vi "1.vi"() -> ()   [LabVIEW 2015]
uses:
  <vilib>/Analysis/NI_AALBase.lvlib
panel:
  out "Simulasi Data":dbl[][](graph)
  in  "UUT Serial Number":string
  in  "Operator Name":string
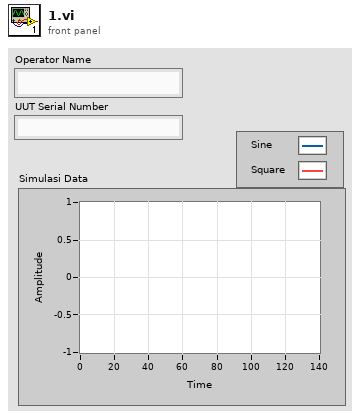
[diagram p1: front panel]
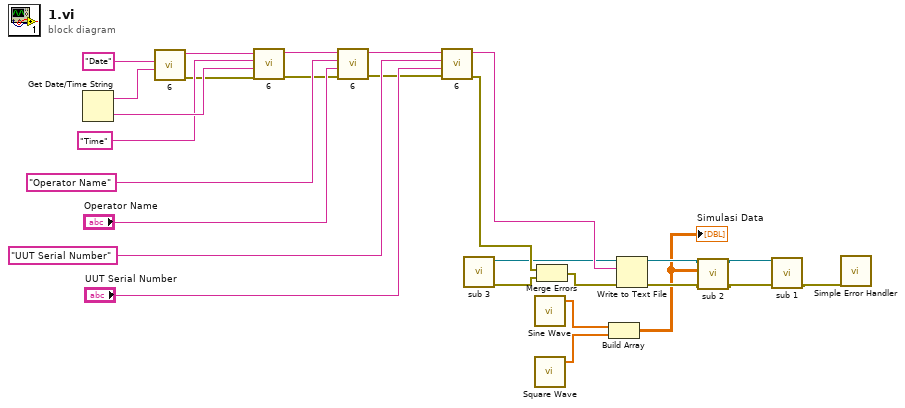
[diagram p0: block diagram]
diagram:
  n1 = Get Date/Time String() -> (date string=w9:string, time string=w8:string)  [unwired: 3 in]
  n2 = call "6.vi"(9:"File Property Name"=w9, 10:"File Property Name"="Date" ("input in")) -> ("error out"=w6:errorcluster, "String out"=w5:string)  [unwired: 8 in]
  n3 = call "6.vi"("error in (no error)"=w6, 9:"File Property Name"=w8, 10:"File Property Name"="Time" ("input in"), "String in"=w5) -> ("error out"=w4:errorcluster, "String out"=w3:string)  [unwired: 6 in]
  n4 = call "6.vi"("error in (no error)"=w4, 9:"File Property Name"="Operator Name", 10:"File Property Name"="Operator Name" ("input in"), "String in"=w3) -> ("error out"=w14:errorcluster, "String out"=w13:string)  [unwired: 6 in]
  n5 = call "6.vi"("error in (no error)"=w14, 9:"File Property Name"="UUT Serial Number", 10:"File Property Name"="UUT Serial Number" ("input 3"), "String in"=w13) -> ("error out"=w18:errorcluster, "String out"=w17:string)  [unwired: 6 in]
  n6 = call "sub 3.vi"() -> ("error out"=w19:errorcluster, "File Refnum Out"=w2:refnum<file>)  [unwired: 10 in]
  n7 = call <vilib>:"Sine Wave.vi"() -> ("sine wave"=w25:dbl[])  [unwired: 5 in, 2 out]
  n8 = call <vilib>:"Square Wave.vi"() -> ("square wave"=w26:dbl[])  [unwired: 6 in, 2 out]
  n9 = Merge Errors(w18, w19) -> (w27:errorcluster)
  n10 = Build Array(w25, w26) -> (w1:dbl[][])
  "Simulasi Data" <- w1
  n11 = Write to Text File(file (use dialog)=w2, text=w17, error in=w27) -> (refnum out=w21:refnum<file>, error out=w20:errorcluster)  [unwired: 1 in, 1 out]
  n12 = call "sub 2.vi"("error in (no error)"=w20, "Data to Log"=w1, "File Refnum In"=w21) -> ("error out"=w23:errorcluster, "File Refnum Out"=w22:refnum<file>)  [unwired: 7 in]
  n13 = call "sub 1.vi"("error in (no error)"=w23, "File Refnum In"=w22) -> ("error out"=w24:errorcluster)  [unwired: 9 in]
  n14 = call <vilib>:"Simple Error Handler.vi"("error in (no error)"=w24) -> ()  [unwired: 4 in, 5 out]
